vi "输出参数设置 - 副本.vi"() -> ()   [LabVIEW 2020]
panel:
  in  "电压下限3":i32(slide) scale=-10.0..1.0
  in  "电压下限1":i32(slide) scale=-10.0..1.0
  in  "VO4对数:":bool
  in  "VO3对数:":bool
  in  "VO2对数:":bool
  in  "VO1对数:":bool
  in  "备注":string
  in  "物理量4下限":dbl=-100.0
  in  "物理量4上限":dbl=100.0
  in  "物理量3下限":dbl=-100.0
  in  "物理量3上限":dbl=100.0
  in  "物理量2下限":dbl=-100.0
  in  "物理量2上限":dbl=100.0
  in  "物理量1下限":dbl=-100.0
  in  "物理量1上限":dbl=100.0
  in  "VO4开关：":bool
  in  "VO3开关：":bool
  in  "VO2开关：":bool
  in  "VO1开关：":bool
  in  "VO4选择：":u16(ring)=3 items=["电流1", "电流1反应性", "电流2", "电流2反应性", "D棒位"]
  in  "VO3选择：":u16(ring)=2 items=["电流1", "电流1反应性", "电流2", "电流2反应性", "D棒位"]
  in  "VO2选择：":u16(ring)=1 items=["电流1", "电流1反应性", "电流2", "电流2反应性", "D棒位"]
  in  "VO1选择：":u16(ring) items=["电流1", "电流1反应性", "电流2", "电流2反应性", "D棒位"]
  in  "电压上限4":i32(slide) scale=1.0..10.0
  in  "电压下限4":i32(slide) scale=-10.0..1.0
  in  "电压上限3":i32(slide) scale=1.0..10.0
  in  "电压上限2":i32(slide) scale=1.0..10.0
  in  "电压下限2":i32(slide) scale=-10.0..1.0
  in  "电压上限1":i32(slide) scale=1.0..10.0
  out "电压标尺8":u16(ring) items=["计数通量", "电压通量", "电流通量", "棒位", "温度", "P2参数", "硼浓度"]
  out "电压标尺7":u16(ring) items=["计数通量", "电压通量", "电流通量", "棒位", "温度", "P2参数", "硼浓度"]
  out "电压标尺6":u16(ring) items=["计数通量", "电压通量", "电流通量", "棒位", "温度", "P2参数", "硼浓度"]
  out "电压标尺5":u16(ring) items=["计数通量", "电压通量", "电流通量", "棒位", "温度", "P2参数", "硼浓度"]
  out "电压标尺4":u16(ring) items=["计数通量", "电压通量", "电流通量", "棒位", "温度", "P2参数", "硼浓度"]
  out "电压标尺3":u16(ring) items=["计数通量", "电压通量", "电流通量", "棒位", "温度", "P2参数", "硼浓度"]
  out "电压标尺2":u16(ring) items=["计数通量", "电压通量", "电流通量", "棒位", "温度", "P2参数", "硼浓度"]
  out "电压标尺1":u16(ring) items=["计数通量", "电压通量", "电流通量", "棒位", "温度", "P2参数", "硼浓度"]
  out "电流2":bool
  out "电流1":bool
  out "电压8":bool
  out "电压7":bool
  out "电压6":bool
  out "电压5":bool
  out "电压4":bool
  in  "恢复":bool caption="Cancel Button"
  out "电压3":bool
  out "电压2":bool
  out "电压1":bool
  out "脉冲3":bool
  out "脉冲2":bool
  out "脉冲1":bool
  in  "取消修改":bool caption="Cancel Button"
  in  "保存修改":bool
  # "输入状态"
  # "输出电压设置"
  # "电流1"
  # "电流2"
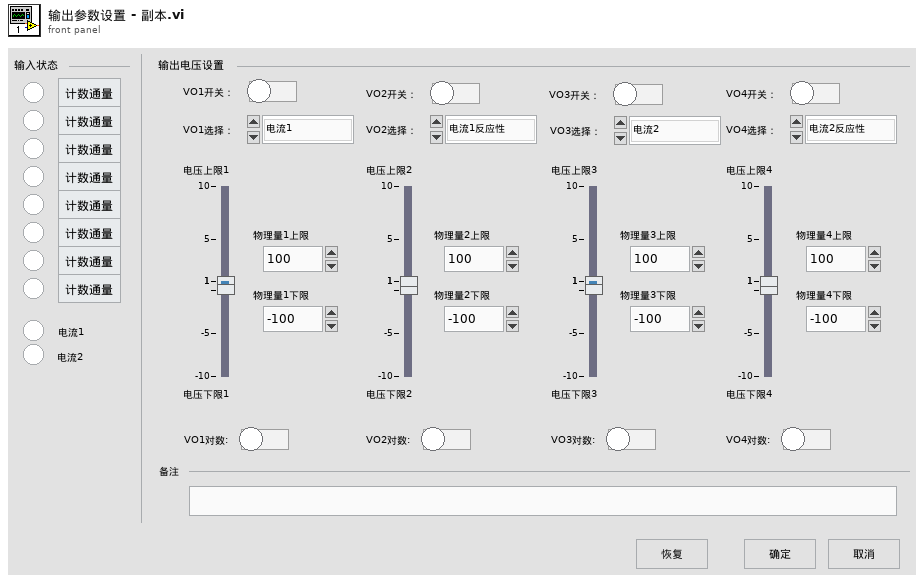
[diagram p1: front panel]
types:
  T1 = enum16{"open", "replace", "create", "open or create", "replace or create", "replace or create with confirmation"}
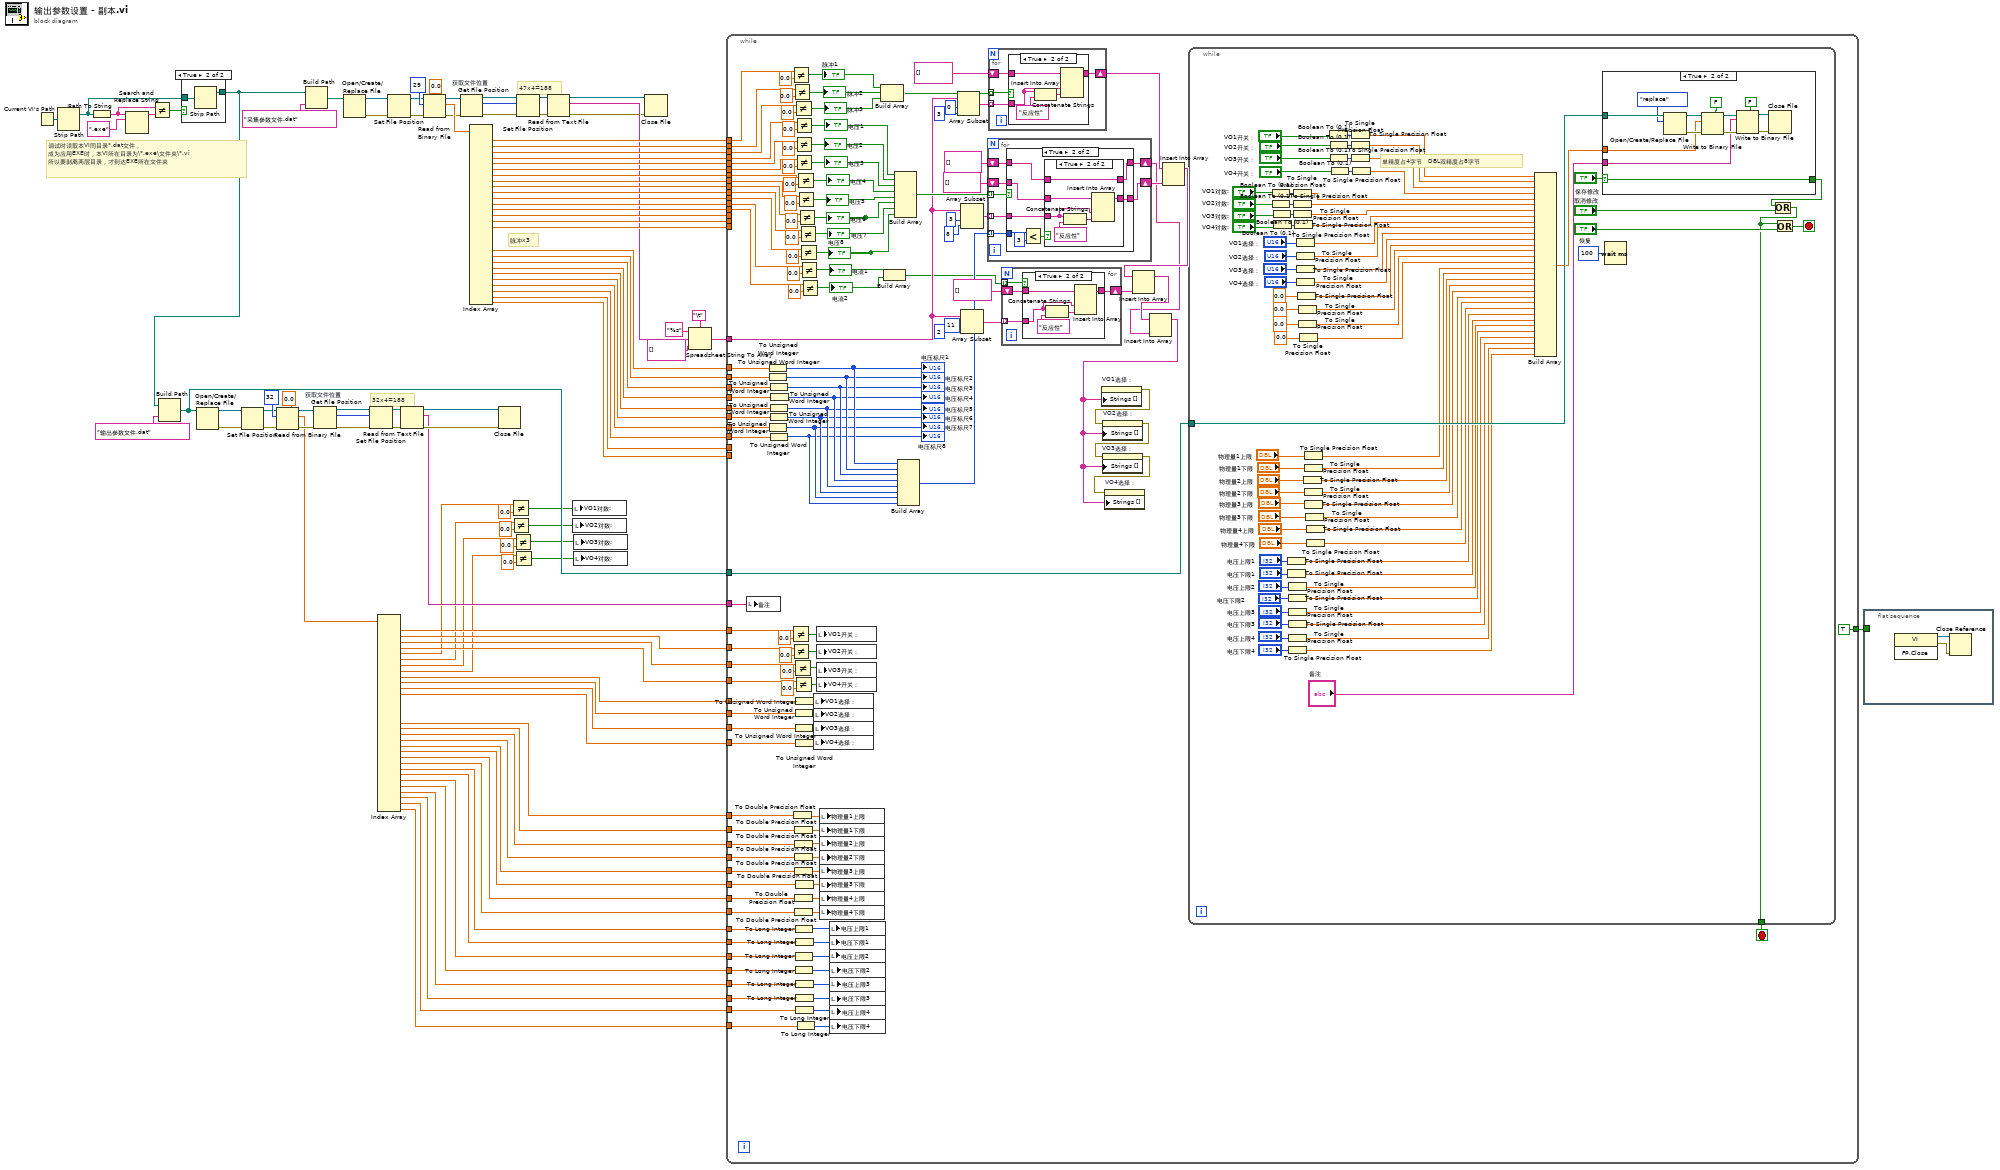
[diagram p0: block diagram]
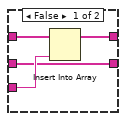
[diagram p6: hidden frame]
diagram:
  # "32x4=188"
  # "调试时读取本VI同目录*.dat文件，\n成为应用EXE时，本VI所在目录为\\*.exe\\文件夹\\*.vi\n所以要剥离两层目录，才到达EXE所在文件夹"
  # "47x4=188"
  # "脉冲x3"
  n1 = Current VI's Path() -> (path=w63:path)
  n2 = Strip Path(path=w63) -> (stripped path=w58:path)  [unwired: 1 out]
  n3 = Path To String(path=w58) -> (string=w60:string)
  n4 = Search and Replace String(input string=w60, search string=".exe" ("搜索字符串")) -> (result string=w61:string)  [unwired: 6 in, 3 out]
  n5 = Not Equal?(x=w60, y=w61) -> (x != y?=w59:bool)
  n6 = case shown="True" w59 {
    tunnel: w58 -> [w113 w115]
    tunnel: [w113 w114] -> w41
    frame False {
    }
    frame True {
      n7 = Strip Path(path=w115) -> (stripped path=w114:path)  [unwired: 1 out]
    }
  }
  n8 = Build Path(base path=w41, name or relative path="输出参数文件.dat") -> (appended path=w35:path)
  n9 = Open/Create/Replace File(file path (use dialog)=w35) -> (refnum out=w50:refnum<file>, error out=w49:errorcluster)  [unwired: 5 in, 1 out]
  n10 = Set File Position(refnum=w50, error in=w49) -> (refnum out=w48:refnum<file>, error out=w47:errorcluster)  [unwired: 2 in]
  n11 = Read from Binary File(5:sgl 0.0 ("byte stream type"), 8:w47, 10:32 ("count"), 11:w48) -> (0:w51:errorcluster, 2:w40:sgl[], 3:w52:refnum<file>)  [unwired: 2 in, 1 out]
  n12 = Build Path(base path=w41, name or relative path="采集参数文件.dat") -> (appended path=w106:path)
  n13 = Get File Position "获取文件位置"(4:w51, 7:w52) -> (0:w54:errorcluster, 2:w42:i64, 3:w55:refnum<file>)
  n14 = Open/Create/Replace File(file path (use dialog)=w106) -> (refnum out=w89:refnum<file>, error out=w88:errorcluster)  [unwired: 5 in, 1 out]
  n15 = Set File Position(offset (in bytes) (0)=w42, refnum=w55, error in=w54) -> (refnum out=w46:refnum<file>, error out=w45:errorcluster)  [unwired: 1 in]
  n16 = Index Array(array=w40) -> (element #1=w39:sgl, element #2=w38:sgl, element #3=w37:sgl, element #4=w36:sgl, element #5=w8:sgl, element #6=w7:sgl, element #7=w6:sgl, element #8=w5:sgl, element #9=w34:sgl, element #10=w33:sgl, element #11=w32:sgl, element #12=w31:sgl, element #17=w30:sgl, element #18=w29:sgl, element #19=w28:sgl, element #20=w27:sgl, element #21=w26:sgl, element #22=w25:sgl, element #23=w24:sgl, element #24=w23:sgl, element #25=w22:sgl, element #26=w21:sgl, element #27=w20:sgl, element #28=w19:sgl, element #29=w18:sgl, element #30=w17:sgl, element #31=w16:sgl, element #32=w15:sgl)  [unwired: 32 in, 4 out]
  n17 = Set File Position(refnum=w89, error in=w88) -> (refnum out=w87:refnum<file>, error out=w86:errorcluster)  [unwired: 2 in]
  n18 = Read from Text File(file (use dialog)=w46, error in=w45) -> (refnum out=w43:refnum<file>, text=w14:string, error out=w44:errorcluster)  [unwired: 1 in, 2 out]
  n19 = Read from Binary File(5:sgl 0.0 ("byte stream type"), 8:w86, 10:29 ("count"), 11:w87) -> (0:w104:errorcluster, 2:w110:sgl[], 3:w105:refnum<file>)  [unwired: 2 in, 1 out]
  n20 = Get File Position "获取文件位置"(4:w104, 7:w105) -> (0:w108:errorcluster, 2:w74:i64, 3:w109:refnum<file>)
  n21 = Index Array(array=w110) -> (element #1=w103:sgl, element #2=w102:sgl, element #3=w101:sgl, element #4=w100:sgl, element #5=w99:sgl, element #6=w98:sgl, element #7=w97:sgl, element #8=w96:sgl, element #9=w95:sgl, element #10=w94:sgl, element #11=w93:sgl, element #12=w92:sgl, element #13=w91:sgl, element #14=w90:sgl, element #15=w85:sgl, element #16=w84:sgl, element #20=w73:sgl, element #21=w72:sgl, element #22=w71:sgl, element #23=w70:sgl, element #24=w69:sgl, element #25=w68:sgl, element #26=w67:sgl, element #27=w66:sgl, element #28=w64:sgl, element #29=w65:sgl)  [unwired: 29 in, 3 out]
  n22 = Close File(refnum=w43, error in=w44) -> ()  [unwired: 2 out]
  n23 = Not Equal?(x=w8, y=sgl 0.0) -> (x != y?=w4:bool)
  n24 = Not Equal?(x=w7, y=sgl 0.0) -> (x != y?=w3:bool)
  n25 = Not Equal?(x=w6, y=sgl 0.0) -> (x != y?=w2:bool)
  n26 = Not Equal?(x=w5, y=sgl 0.0) -> (x != y?=w1:bool)
  n27 = Set File Position(offset (in bytes) (0)=w74, refnum=w109, error in=w108) -> (refnum out=w81:refnum<file>, error out=w80:errorcluster)  [unwired: 1 in]
  n28 = Read from Text File(file (use dialog)=w81, error in=w80) -> (refnum out=w76:refnum<file>, text=w79:string, error out=w77:errorcluster)  [unwired: 1 in, 2 out]
  n29 = local write "VO1对数:"(w4) -> ()
  n30 = local write "VO2对数:"(w3) -> ()
  n31 = local write "VO3对数:"(w2) -> ()
  n32 = local write "VO4对数:"(w1) -> ()
  n33 = Close File(refnum=w76, error in=w77) -> ()  [unwired: 2 out]
  n34 = Spreadsheet String To Array(delimiter (Tab)="\t", format string="%s", spreadsheet string=w79, array type (2D Dbl)=string[] [] ("添加的数组")) -> (array=w75:string[])
  n35 = while {
    tunnel: w103 -> [w254]
    tunnel: w102 -> [w249]
    tunnel: w101 -> [w248]
    tunnel: w100 -> [w247]
    tunnel: w99 -> [w244]
    tunnel: w98 -> [w242]
    tunnel: w97 -> [w236]
    tunnel: w96 -> [w235]
    tunnel: w95 -> [w234]
    tunnel: w94 -> [w233]
    tunnel: w93 -> [w232]
    tunnel: w92 -> [w229]
    tunnel: w91 -> [w228]
    tunnel: w90 -> [_]
    tunnel: w85 -> [_]
    tunnel: w84 -> [_]
    tunnel: w75 -> [w136]
    tunnel: w73 -> [w227]
    tunnel: w72 -> [w226]
    tunnel: w71 -> [w225]
    tunnel: w70 -> [w224]
    tunnel: w69 -> [w223]
    tunnel: w68 -> [w222]
    tunnel: w67 -> [w221]
    tunnel: w66 -> [w220]
    tunnel: w64 -> [_]
    tunnel: w65 -> [_]
    tunnel: w39 -> [w198]
    tunnel: w38 -> [w197]
    tunnel: w37 -> [w196]
    tunnel: w36 -> [w195]
    tunnel: w35 -> [w194]
    tunnel: w34 -> [w165]
    tunnel: w33 -> [w164]
    tunnel: w32 -> [w163]
    tunnel: w31 -> [w162]
    tunnel: w30 -> [w161]
    tunnel: w29 -> [w160]
    tunnel: w28 -> [w159]
    tunnel: w27 -> [w158]
    tunnel: w26 -> [w157]
    tunnel: w25 -> [w156]
    tunnel: w24 -> [w155]
    tunnel: w23 -> [w154]
    tunnel: w22 -> [w153]
    tunnel: w21 -> [w152]
    tunnel: w20 -> [w151]
    tunnel: w19 -> [w150]
    tunnel: w18 -> [w149]
    tunnel: w17 -> [w148]
    tunnel: w16 -> [w147]
    tunnel: w15 -> [w146]
    tunnel: w14 -> [w121]
    tunnel: [TRUE ("子VI退出")] -> w13
    stop <- w246 stop-if-true
    n36 = local write "备注"(w121) -> ()
    n37 = To Unsigned Word Integer(number=w227) -> (unsigned 16bit integer=w193:u16)
    "电压标尺1" <- w193
    n38 = To Unsigned Word Integer(number=w226) -> (unsigned 16bit integer=w192:u16)
    "电压标尺2" <- w192
    n39 = To Unsigned Word Integer(number=w221) -> (unsigned 16bit integer=w187:u16)
    "电压标尺7" <- w187
    n40 = To Unsigned Word Integer(number=w225) -> (unsigned 16bit integer=w191:u16)
    "电压标尺3" <- w191
    n41 = To Unsigned Word Integer(number=w223) -> (unsigned 16bit integer=w189:u16)
    "电压标尺5" <- w189
    n42 = To Unsigned Word Integer(number=w222) -> (unsigned 16bit integer=w188:u16)
    "电压标尺6" <- w188
    n43 = To Unsigned Word Integer(number=w220) -> (unsigned 16bit integer=w186:u16)
    "电压标尺8" <- w186
    n44 = To Unsigned Word Integer(number=w224) -> (unsigned 16bit integer=w190:u16)
    "电压标尺4" <- w190
    n45 = Not Equal?(x=w198, y=sgl 0.0) -> (x != y?=w120:bool)
    n46 = Not Equal?(x=w254, y=sgl 0.0) -> (x != y?=w212:bool)
    "脉冲1" <- w212
    n47 = Not Equal?(x=w197, y=sgl 0.0) -> (x != y?=w119:bool)
    n48 = Not Equal?(x=w249, y=sgl 0.0) -> (x != y?=w211:bool)
    "脉冲2" <- w211
    n49 = Not Equal?(x=w196, y=sgl 0.0) -> (x != y?=w118:bool)
    n50 = To Double Precision Float(number=w161) -> (double precision float=w181:dbl)
    n51 = Not Equal?(x=w248, y=sgl 0.0) -> (x != y?=w210:bool)
    "脉冲3" <- w210
    n52 = Not Equal?(x=w195, y=sgl 0.0) -> (x != y?=w117:bool)
    n53 = To Unsigned Word Integer(number=w164) -> (unsigned 16bit integer=w184:u16)
    n54 = To Unsigned Word Integer(number=w163) -> (unsigned 16bit integer=w183:u16)
    n55 = To Double Precision Float(number=w160) -> (double precision float=w180:dbl)
    n56 = To Double Precision Float(number=w159) -> (double precision float=w179:dbl)
    n57 = To Double Precision Float(number=w158) -> (double precision float=w178:dbl)
    n58 = To Double Precision Float(number=w157) -> (double precision float=w177:dbl)
    n59 = To Double Precision Float(number=w155) -> (double precision float=w175:dbl)
    n60 = To Double Precision Float(number=w154) -> (double precision float=w174:dbl)
    n61 = To Long Integer(number=w153) -> (32bit integer=w173:i32)
    n62 = To Long Integer(number=w151) -> (32bit integer=w171:i32)
    n63 = To Long Integer(number=w150) -> (32bit integer=w170:i32)
    n64 = Not Equal?(x=w247, y=sgl 0.0) -> (x != y?=w144:bool)
    "电压1" <- w144
    n65 = Not Equal?(x=w244, y=sgl 0.0) -> (x != y?=w219:bool)
    "电压2" <- w219
    n66 = Not Equal?(x=w242, y=sgl 0.0) -> (x != y?=w218:bool)
    "电压3" <- w218
    n67 = To Unsigned Word Integer(number=w165) -> (unsigned 16bit integer=w185:u16)
    n68 = To Unsigned Word Integer(number=w162) -> (unsigned 16bit integer=w182:u16)
    n69 = To Double Precision Float(number=w156) -> (double precision float=w176:dbl)
    n70 = To Long Integer(number=w152) -> (32bit integer=w172:i32)
    n71 = To Long Integer(number=w149) -> (32bit integer=w169:i32)
    n72 = To Long Integer(number=w148) -> (32bit integer=w168:i32)
    n73 = To Long Integer(number=w147) -> (32bit integer=w167:i32)
    n74 = Not Equal?(x=w236, y=sgl 0.0) -> (x != y?=w217:bool)
    "电压4" <- w217
    n75 = To Long Integer(number=w146) -> (32bit integer=w166:i32)
    n76 = Not Equal?(x=w235, y=sgl 0.0) -> (x != y?=w216:bool)
    "电压5" <- w216
    n77 = Not Equal?(x=w234, y=sgl 0.0) -> (x != y?=w215:bool)
    "电压6" <- w215
    n78 = Not Equal?(x=w233, y=sgl 0.0) -> (x != y?=w214:bool)
    "电压7" <- w214
    n79 = Not Equal?(x=w232, y=sgl 0.0) -> (x != y?=w213:bool)
    "电压8" <- w213
    n80 = Not Equal?(x=w229, y=sgl 0.0) -> (x != y?=w205:bool)
    "电流1" <- w205
    n81 = Not Equal?(x=w228, y=sgl 0.0) -> (x != y?=w204:bool)
    "电流2" <- w204
    n82 = local write "VO1选择："(w185) -> ()
    n83 = local write "VO2选择："(w184) -> ()
    n84 = local write "VO3选择："(w183) -> ()
    n85 = local write "VO4选择："(w182) -> ()
    n86 = local write "VO1开关："(w120) -> ()
    n87 = local write "VO2开关："(w119) -> ()
    n88 = local write "VO3开关："(w118) -> ()
    n89 = local write "VO4开关："(w117) -> ()
    n90 = local write "物理量1上限"(w181) -> ()
    n91 = local write "物理量1下限"(w180) -> ()
    n92 = local write "物理量2上限"(w179) -> ()
    n93 = local write "物理量2下限"(w178) -> ()
    n94 = local write "物理量3上限"(w177) -> ()
    n95 = local write "物理量3下限"(w176) -> ()
    n96 = local write "物理量4上限"(w175) -> ()
    n97 = local write "物理量4下限"(w174) -> ()
    n98 = local write "电压上限1"(w173) -> ()
    n99 = local write "电压下限1"(w172) -> ()
    n100 = local write "电压上限2"(w171) -> ()
    n101 = local write "电压下限2"(w170) -> ()
    n102 = local write "电压上限3"(w169) -> ()
    n103 = local write "电压下限3"(w168) -> ()
    n104 = local write "电压上限4"(w167) -> ()
    n105 = local write "电压下限4"(w166) -> ()
    n106 = Build Array(w212, w211, w210) -> (w209:bool[])
    n107 = Build Array(w205, w204) -> (w135:bool[])
    n108 = Build Array(w144, w219, w218, w217, w216, w215, w214, w213) -> (w206:bool[])
    n109 = Build Array(w193, w192, w191, w190, w189, w188, w187, w186) -> (w203:u16[])
    n110 = Array Subset(array=w136, index=0 ("索引"), length=3 ("长度")) -> (w141:string[])
    n111 = Array Subset(array=w136, index=3 ("索引"), length=8 ("长度")) -> (w207:string[])
    n112 = Array Subset(array=w136, index=11 ("索引"), length=2 ("长度")) -> (w134:string[])
    n113 = for {
      tunnel: w207 -> [w277] mode=indexing
      tunnel: w206 -> [w281] mode=indexing
      tunnel: w203 -> [w279] mode=indexing
      shift-right: [w278] -> w131
      shift-left: string[] [] ("子数组") -> [w280]
      shift-right: [w275] -> w122
      shift-left: string[] [] ("子数组") -> [w276]
      n114 = case shown="True" w281 {
        tunnel: w280 -> [w283 w288]
        tunnel: w279 -> [_ w291]
        tunnel: [w283 w287] -> w278
        tunnel: w277 -> [_ w286]
        tunnel: w276 -> [w282 w284]
        tunnel: [w282 w285] -> w275
        frame False {
        }
        frame True {
          n115 = Less?(x=w291, y=u16 3) -> (x < y?=w289:bool)
          n116 = case shown="True" w289 {
            tunnel: w288 -> [w292 w299]
            tunnel: [w292 w298] -> w287
            tunnel: w286 -> [w295 w297]
            tunnel: [w293 w296] -> w285
            tunnel: w284 -> [w294 w296]
            frame False {
              n117 = Insert Into Array(array=w294, new element=w295) -> (w293:string[])  [unwired: 1 in]
            }
            frame True {
              n118 = Concatenate Strings(w297, "反应性" ("字符串")) -> (w300:string)
              n119 = Insert Into Array(array=w299, new element #1=w297, new element #2=w300) -> (w298:string[])  [unwired: 1 in]
            }
          }
        }
      }
    }
    n120 = for {
      tunnel: w209 -> [w266] mode=indexing
      tunnel: w141 -> [w265] mode=indexing
      shift-right: [w267] -> w132
      shift-left: string[] [] ("子数组") -> [w268]
      n121 = case shown="True" w266 {
        tunnel: w268 -> [w269 w274]
        tunnel: [w269 w273] -> w267
        tunnel: w265 -> [_ w272]
        frame False {
        }
        frame True {
          n122 = Concatenate Strings(w272, "反应性" ("字符串")) -> (w270:string)
          n123 = Insert Into Array(array=w274, new element #1=w272, new element #2=w270) -> (w273:string[])  [unwired: 1 in]
        }
      }
    }
    n124 = for {
      tunnel: w135 -> [w256] mode=indexing
      tunnel: w134 -> [w255] mode=indexing
      shift-right: [w257] -> w129
      shift-left: string[] [] ("子数组") -> [w258]
      n125 = case shown="True" w256 {
        tunnel: w258 -> [w259 w264]
        tunnel: [w259 w263] -> w257
        tunnel: w255 -> [_ w260]
        frame False {
        }
        frame True {
          n126 = Concatenate Strings(w260, "反应性" ("字符串")) -> (w261:string)
          n127 = Insert Into Array(array=w264, new element #1=w260, new element #2=w261) -> (w263:string[])  [unwired: 1 in]
        }
      }
    }
    n128 = Insert Into Array(array=w132, new element=w131) -> (w130:string[])  [unwired: 1 in]
    n129 = Insert Into Array(array=w130, new element=w129) -> (w124:string[])  [unwired: 1 in]
    n130 = Insert Into Array(array=w124, new element=w122) -> (w123:string[])  [unwired: 1 in]
    n131 = property on="VO1选择：" class="Ring (strict)"("Strings []"=w123) -> (error out=w128:errorcluster)  [unwired: 2 in, 1 out]
    n132 = property on="VO2选择：" class="Ring (strict)"(error in=w128, "Strings []"=w123) -> (error out=w127:errorcluster)  [unwired: 1 in, 1 out]
    n133 = property on="VO3选择：" class="Ring (strict)"(error in=w127, "Strings []"=w123) -> (error out=w126:errorcluster)  [unwired: 1 in, 1 out]
    n134 = property on="VO4选择：" class="Ring (strict)"(error in=w126, "Strings []"=w123) -> ()  [unwired: 1 in, 2 out]
    n135 = while {
      tunnel: w194 -> [w383]
      tunnel: [w370] -> w246
      stop <- w371 stop-if-true
      # "单精度占4字节   DBL双精度占8字节"
      n136 = Boolean To (0,1)(Boolean="VO1对数:") -> (0, 1=w378:i16)
      n137 = Boolean To (0,1)(Boolean="VO2对数:") -> (0, 1=w377:i16)
      n138 = Boolean To (0,1)(Boolean="VO3对数:") -> (0, 1=w368:i16)
      n139 = Boolean To (0,1)(Boolean="VO4对数:") -> (0, 1=w369:i16)
      n140 = To Single Precision Float(number="电压上限1") -> (single precision float=w318:sgl)
      n141 = To Single Precision Float(number="电压下限1") -> (single precision float=w317:sgl)
      n142 = To Single Precision Float(number="电压上限2") -> (single precision float=w316:sgl)
      n143 = To Single Precision Float(number="电压下限2") -> (single precision float=w315:sgl)
      n144 = To Single Precision Float(number="电压上限3") -> (single precision float=w314:sgl)
      n145 = To Single Precision Float(number="电压上限4") -> (single precision float=w312:sgl)
      n146 = To Single Precision Float(number="电压下限4") -> (single precision float=w311:sgl)
      n147 = To Single Precision Float(number="电压下限3") -> (single precision float=w313:sgl)
      n148 = To Single Precision Float(number=w378) -> (single precision float=w331:sgl)
      n149 = To Single Precision Float(number=w377) -> (single precision float=w333:sgl)
      n150 = To Single Precision Float(number=w368) -> (single precision float=w334:sgl)
      n151 = To Single Precision Float(number=w369) -> (single precision float=w335:sgl)
      n152 = To Single Precision Float(number="VO1选择：") -> (single precision float=w336:sgl)
      n153 = To Single Precision Float(number="VO2选择：") -> (single precision float=w337:sgl)
      n154 = To Single Precision Float(number="VO3选择：") -> (single precision float=w338:sgl)
      n155 = To Single Precision Float(number="VO4选择：") -> (single precision float=w339:sgl)
      n156 = To Single Precision Float(number=sgl 0.0 ("数字")) -> (single precision float=w340:sgl)
      n157 = To Single Precision Float(number=sgl 0.0 ("数字")) -> (single precision float=w341:sgl)
      n158 = To Single Precision Float(number=sgl 0.0 ("数字")) -> (single precision float=w342:sgl)
      n159 = To Single Precision Float(number=sgl 0.0 ("数字")) -> (single precision float=w343:sgl)
      n160 = To Single Precision Float(number="物理量2上限") -> (single precision float=w324:sgl)
      n161 = To Single Precision Float(number="物理量1上限") -> (single precision float=w326:sgl)
      n162 = To Single Precision Float(number="物理量1下限") -> (single precision float=w325:sgl)
      n163 = To Single Precision Float(number="物理量2下限") -> (single precision float=w323:sgl)
      n164 = To Single Precision Float(number="物理量3上限") -> (single precision float=w322:sgl)
      n165 = To Single Precision Float(number="物理量3下限") -> (single precision float=w321:sgl)
      n166 = To Single Precision Float(number="物理量4上限") -> (single precision float=w320:sgl)
      n167 = To Single Precision Float(number="物理量4下限") -> (single precision float=w319:sgl)
      n168 = Boolean To (0,1)(Boolean="VO1开关：") -> (0, 1=w382:i16)
      n169 = Boolean To (0,1)(Boolean="VO2开关：") -> (0, 1=w381:i16)
      n170 = Boolean To (0,1)(Boolean="VO3开关：") -> (0, 1=w380:i16)
      n171 = Boolean To (0,1)(Boolean="VO4开关：") -> (0, 1=w379:i16)
      n172 = To Single Precision Float(number=w382) -> (single precision float=w327:sgl)
      n173 = To Single Precision Float(number=w381) -> (single precision float=w328:sgl)
      n174 = To Single Precision Float(number=w380) -> (single precision float=w329:sgl)
      n175 = To Single Precision Float(number=w379) -> (single precision float=w330:sgl)
      n176 = Build Array(w327, w328, w329, w330, w331, w333, w334, w335, w336, w337, w338, w339, w340, w341, w342, w343, w326, w325, w324, w323, w322, w321, w320, w319, w318, w317, w316, w315, w314, w313, w312, w311) -> (w332:sgl[])
      n177 = case shown="True" "保存修改" {
        selector: "保存修改" -> [w384 w391]
        tunnel: w383 -> [_ w397]
        tunnel: w332 -> [_ w393]
        tunnel: [w384 w391] -> w375
        tunnel: "备注" -> [_ w385]
        frame False {
        }
        frame True {
          n178 = Open/Create/Replace File(file path (use dialog)=w397, operation (0:open)=T1."replace" ("操作(0:open)")) -> (refnum out=w396:refnum<file>, error out=w395:errorcluster)  [unwired: 4 in, 1 out]
          n179 = Write to Binary File(file (use dialog)=w396, data=w393, error in=w395, 5:FALSE ("预置数组或字符串大小？(T)")) -> (refnum out=w388:refnum<file>, error out=w390:errorcluster)  [unwired: 2 in, 1 out]
          n180 = Write to Binary File(file (use dialog)=w388, data=w385, error in=w390, 5:FALSE ("预置数组或字符串大小？(T)")) -> (refnum out=w387:refnum<file>, error out=w389:errorcluster)  [unwired: 2 in, 1 out]
          n181 = Close File(refnum=w387, error in=w389) -> ()  [unwired: 2 out]
        }
      }
      n182 = Wait (ms)(milliseconds to wait=u32 100 ("等待时间（毫秒）")) -> ()  [unwired: 1 out]
      n183 = Or(x=w375, y="取消修改") -> (x .or. y?=w370:bool)
      n184 = Or(x=w370, y="恢复") -> (x .or. y?=w371:bool)
    }
  }
  n185 = flat-sequence {
    tunnel: w13 -> [_]
    frame #0 {
      n186 = invoke class="VI" method="FP.Close"() -> (reference out=w398:refnum<vi>, error out=w399:errorcluster)  [unwired: 3 in, 1 out]
      n187 = Close Reference(reference=w398, error in (no error)=w399) -> ()  [unwired: 1 out]
    }
  }
